vi "HIOKI PW3390 Continuous Acquisition Plot.vi"() -> ()   [LabVIEW 2009]
doc: "Continues to output and plot the specified measurement data in 100ms cycle."
uses:
  <instrlib>/PW3390/Common/_Initialize/HIOKI PW3390 Initialize LAN.vi
  <instrlib>/PW3390/Common/_Initialize/HIOKI PW3390 Initialize RS-232C.vi
panel:
  in  "Item":T1(array[cluster])=[{"Item"=enum."Urms", "Ch(0:Ch1)"=enum."1"}, {"Item"=enum."Urms", "Ch(0:Ch1)"=enum."2"}, {"Item"=enum."Urms", "Ch(0:Ch1)"=enum."3"}, {"Item"=enum."Urms", "Ch(0:Ch1)"=enum."4"}]
  out "error out":errorcluster
  in  "Communication Interface":enum16{"LAN", "RS-232C"}(ring)
  in  "COM Port":refnum<visa-resource-name>="COM1"
  in  "baud rate (38400bps)":u32=38400
  in  "IP Address":string="192.168.1.1"
  out "Data out":dbl[](array[numeric])
  out "4th data":dbl(graph)
  out "3rd data":dbl(graph)
  out "2nd data":dbl(graph)
  out "1st data":dbl(graph)
  in  "Stop":bool
  # "1st"
  # "2nd"
  # "3rd"
  # "4th"
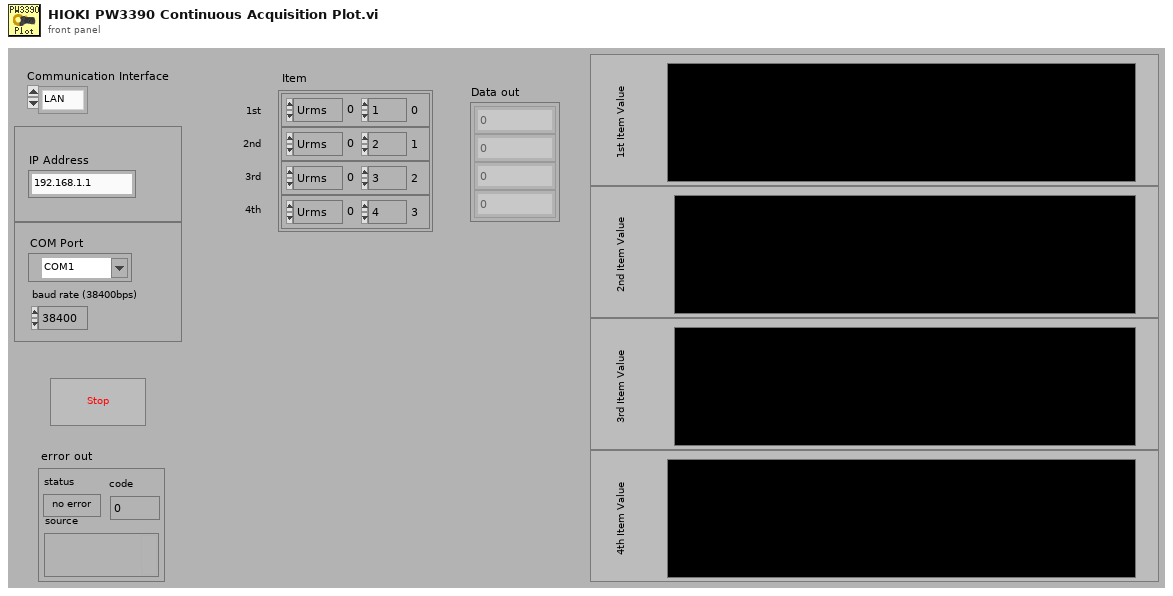
[diagram p1: front panel]
types:
  T1 = cluster{"Item":enum16{"Urms", "Umn", "Uac", "Udc", "Ufnd", "Upk+", "Upk-", "Uthd", "Urf", "Uunb", "Irms", "Imn", "Iac", "Idc", "Ifnd", "Ipk+", "Ipk-", "Ithd", "Irf", "Iunb", "P", "S", "Q", "PF", "DEG U", "DEG I", "DEG P", "f", "EFFI", "LOSS", "IH+", "IH-", "IH", "WP+", "WP-", "WP", "CH A", "CH B", "Pm", "Slip", "Laptime", "Laptime(ms)"}, "Ch(0:Ch1)":enum16{"1", "2", "3", "4", "12", "34", "123"}}[]
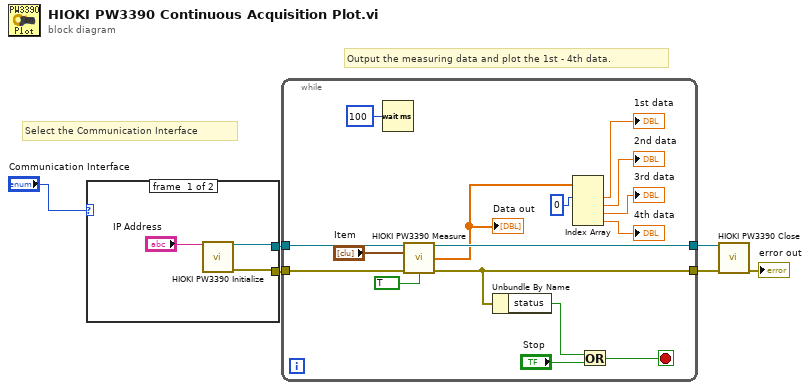
[diagram p0: block diagram]
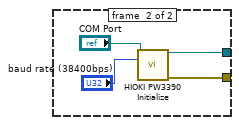
[diagram p2: hidden frame]
diagram:
  # "Select the Communication Interface"
  # "Output the measuring data and plot the 1st - 4th data."
  n1 = case shown="\"LAN\", デフォルト" "Communication Interface" {
    tunnel: [w8 w13] -> w3
    tunnel: [w7 w12] -> w2
    frame #0 {
      n2 = call-poly <instrlib>:"HIOKI PW3390 Initialize.vi"("IP Address"="IP Address") -> ("VISA Resource out"=w8:refnum<visa-resource-name>, "error out"=w7:errorcluster)  [unwired: 12 in, 1 out]
    }
    frame #1 {
      n3 = call-poly <instrlib>:"HIOKI PW3390 Initialize.vi"("COM Port"="COM Port", "baud rate (38400bps)"="baud rate (38400bps)") -> ("VISA Resource out"=w13:refnum<visa-resource-name>, "error out"=w12:errorcluster)  [unwired: 11 in, 1 out]
    }
  }
  n4 = while {
    tunnel: w3 -> [w29]
    tunnel: w2 -> [w28]
    tunnel: [w27] -> w6
    tunnel: [w26] -> w5
    stop <- w23 stop-if-true
    n5 = Wait (ms)(milliseconds to wait=u32 100) -> ()  [unwired: 1 out]
    n6 = call <instrlib>:"HIOKI PW3390 Measure.vi"("VISA Resource"=w29, "Item"="Item", "error in (no error)"=w28, "Error Out (F: Off)"=TRUE) -> ("VISA Resource out"=w27:refnum<visa-resource-name>, "Data out"=w22:dbl[], "error out"=w26:errorcluster)  [unwired: 6 in, 3 out]
    "Data out" <- w22
    n7 = Unbundle By Name(w26) -> ("status"=w24:bool)
    n8 = Index Array(array=w22, index #1=0 ("指標")) -> (element #1=→"1st data":dbl, element #2=→"2nd data":dbl, element #3=→"3rd data":dbl, element #4=→"4th data":dbl)  [unwired: 3 in]
    n9 = Or(x=w24, y="Stop") -> (x .or. y?=w23:bool)
  }
  n10 = call <instrlib>:"HIOKI PW3390 Close.vi"("VISA Resource"=w6, "error in (no error)"=w5) -> ("error out"=→"error out":errorcluster)  [unwired: 13 in]
